vi "pump control trial.vi"(2 "Set standby speed":bool, 4 "Standby/Full speed":bool, 5 "Set standby speed":dbl=20.0 min=20.0 max=30.0 step=0.3000030517578125 format="%#.1f", 7 "VISA resource name":refnum<visa-resource-name>, 8 "Turn On/Off":bool) -> (0 "Pump controller temperature":dbl, 1 "Pump temperature":dbl, 3 "Speed":dbl, 6 "% full speed":i8)   [LabVIEW 2016]
uses:
  <vilib>/Instr/_visa.llb/VISA Configure Serial Port (Instr).vi
panel:
  out "error out 4":errorcluster
  out "error out 3":errorcluster
  out "error out":errorcluster
  out "on feedback":string
  out "off feedback":string
  out "set stb feedback":string
  out "stanby conf":string
  out "full conf":string
  out "error out 2":errorcluster
  out "Standby/Full speed 2":bool
  out "temperature feedback":string
  out "Running speed":string
  in  "baud rate (9600)":u32=9600
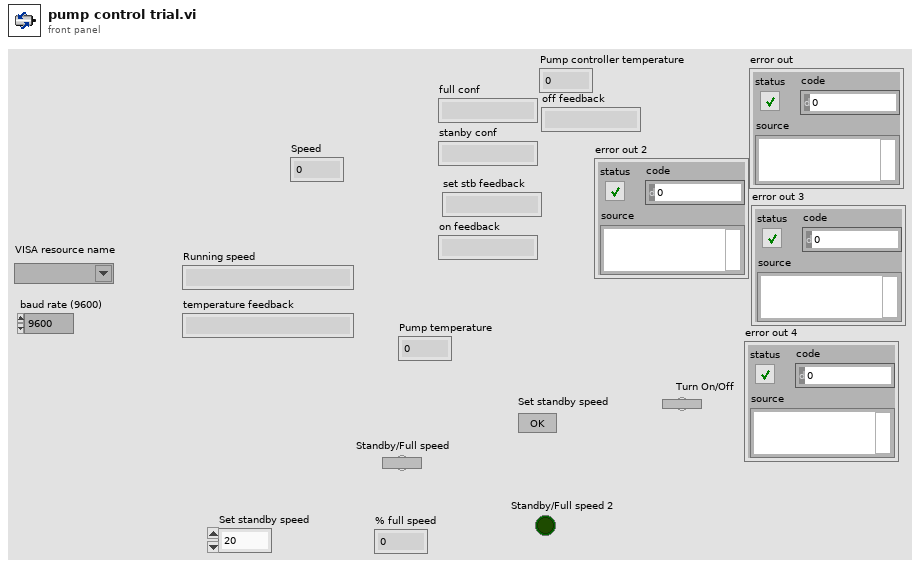
[diagram p1: front panel]
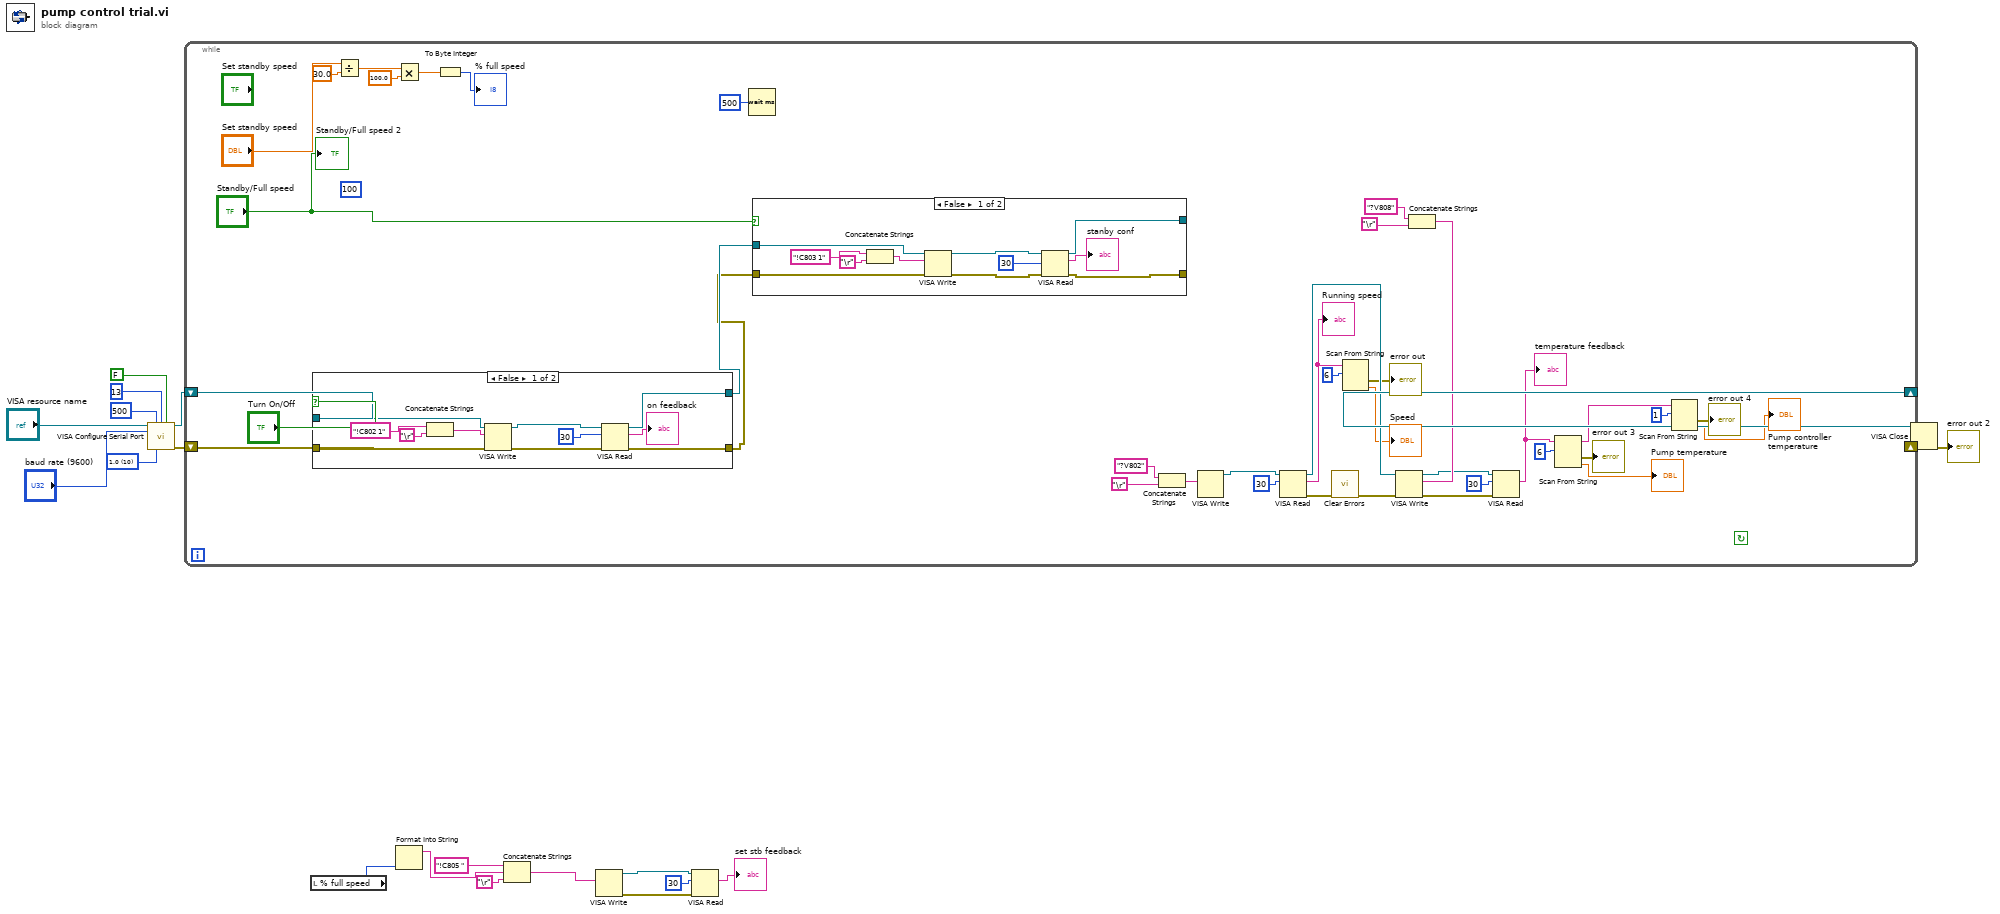
[diagram p0: block diagram]
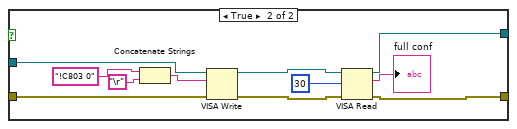
[diagram p2: hidden frame]
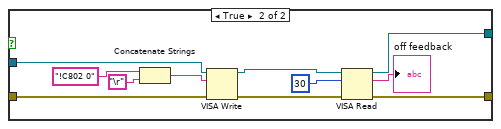
[diagram p3: hidden frame]
diagram:
  w18 = u16 10 items=["1.0"=10, "1.5"=15, "2.0"=20] ("stop bits (10: 1 bit)")
  n1 = call-poly "VISA Configure Serial Port"("VISA resource name"="VISA resource name", "timeout (10sec)"=u32 500, "termination char\n(0xA = '\\n' = LF)"=u8 13 ("termination char\n(0xA = '\\n' = LF)"), "Enable Termination\nChar (T)"=FALSE ("Enable Termination\nChar (T)"), "baud rate (9600)"="baud rate (9600)", "stop bits (10: 1 bit)"=w18) -> ("VISA resource name out"=w17:refnum<visa-resource-name>, "error out"=w16:errorcluster)  [unwired: 8 in]
  n2 = while {
    shift-right: [w61] -> w14
    shift-left: w17 -> [w28]
    shift-right: [w62] -> w13
    shift-left: w16 -> [w27]
    stop <- _ continue-if-true
    (unwired) 100
    n3 = case shown="False" "Turn On/Off" {
      tunnel: w28 -> [w99 w112]
      tunnel: w27 -> [w98 w110]
      tunnel: [w92 w108] -> w24
      tunnel: [w97 w107] -> w25
      frame False {
        n4 = Concatenate Strings("!C802 1" ("string"), "\r" ("string")) -> (w94:string)
        n5 = VISA Write(VISA resource name=w99, write buffer=w94, error in (no error)=w98) -> (VISA resource name out=w101:refnum<visa-resource-name>, error out=w100:errorcluster)  [unwired: 1 out]
        n6 = VISA Read(VISA resource name=w101, byte count=u32 30, error in (no error)=w100) -> (VISA resource name out=w97:refnum<visa-resource-name>, read buffer=→"on feedback":string, error out=w92:errorcluster)  [unwired: 1 out]
      }
      frame True {
        n7 = Concatenate Strings("!C802 0" ("string"), "\r" ("string")) -> (w104:string)
        n8 = VISA Write(VISA resource name=w112, write buffer=w104, error in (no error)=w110) -> (VISA resource name out=w111:refnum<visa-resource-name>, error out=w109:errorcluster)  [unwired: 1 out]
        n9 = VISA Read(VISA resource name=w111, byte count=u32 30, error in (no error)=w109) -> (VISA resource name out=w107:refnum<visa-resource-name>, read buffer=→"off feedback":string, error out=w108:errorcluster)  [unwired: 1 out]
      }
    }
    n10 = Divide(x="Set standby speed", y=30.0) -> (x/y=w64:dbl)
    n11 = Multiply(x=w64, y=sgl 100.0) -> (x*y=w67:dbl)
    n12 = To Byte Integer(number=w67) -> (8bit integer=→"% full speed":i8)
    n13 = Wait (ms)(milliseconds to wait=u32 500) -> ()  [unwired: 1 out]
    n14 = case shown="False" "Standby/Full speed" {
      tunnel: w25 -> [w76 w86]
      tunnel: w24 -> [w78 w85]
      tunnel: [w77 w84] -> _
      tunnel: [w74 w83] -> _
      frame False {
        n15 = Concatenate Strings("!C803 1" ("string"), "\r") -> (w73:string)
        n16 = VISA Write(VISA resource name=w76, write buffer=w73, error in (no error)=w78) -> (VISA resource name out=w75:refnum<visa-resource-name>, error out=w79:errorcluster)  [unwired: 1 out]
        n17 = VISA Read(VISA resource name=w75, byte count=u32 30, error in (no error)=w79) -> (VISA resource name out=w74:refnum<visa-resource-name>, read buffer=→"stanby conf":string, error out=w77:errorcluster)  [unwired: 1 out]
      }
      frame True {
        n18 = Concatenate Strings("!C803 0" ("string"), "\r") -> (w88:string)
        n19 = VISA Write(VISA resource name=w86, write buffer=w88, error in (no error)=w85) -> (VISA resource name out=w89:refnum<visa-resource-name>, error out=w90:errorcluster)  [unwired: 1 out]
        n20 = VISA Read(VISA resource name=w89, byte count=u32 30, error in (no error)=w90) -> (VISA resource name out=w83:refnum<visa-resource-name>, read buffer=→"full conf":string, error out=w84:errorcluster)  [unwired: 1 out]
      }
    }
    n21 = Concatenate Strings("?V802" ("write buffer"), "\r") -> (w52:string)
    n22 = VISA Write(write buffer=w52) -> (VISA resource name=w58:refnum<visa-resource-name>, error in (no error)=w59:errorcluster, VISA resource name out=w53:refnum<visa-resource-name>)  [unwired: 2 out]
    n23 = VISA Read(VISA resource name=w53, byte count=u32 30) -> (VISA resource name out=w55:refnum<visa-resource-name>, read buffer=w36:string, error out=w44:errorcluster)  [unwired: 1 in, 1 out]
    "Running speed" <- w36
    n24 = call <vilib>:"Clear Errors.vi"("error in (no error)"=w44) -> ("error out"=w33:errorcluster)  [unwired: 5 in, 1 out]
    n25 = Scan From String(input string=w36, initial scan location=u32 6) -> (error out=→"error out":errorcluster, output 1=→"Speed":dbl)  [unwired: 3 in, 2 out]
    n26 = Concatenate Strings("?V808" ("write buffer"), "\r") -> (w47:string)
    n27 = VISA Write(VISA resource name=w55, write buffer=w47, error in (no error)=w33) -> (VISA resource name out=w46:refnum<visa-resource-name>, error out=w43:errorcluster)  [unwired: 1 out]
    n28 = VISA Read(VISA resource name=w46, byte count=u32 30, error in (no error)=w43) -> (VISA resource name out=w56:refnum<visa-resource-name>, read buffer=w42:string, error out=w57:errorcluster)  [unwired: 1 out]
    "temperature feedback" <- w42
    n29 = Scan From String(input string=w42, initial scan location=u32 6) -> (remaining string=w39:string, error out=→"error out 3":errorcluster, output 1=→"Pump temperature":dbl)  [unwired: 3 in, 1 out]
    n30 = Scan From String(input string=w39, initial scan location=u32 1) -> (error out=→"error out 4":errorcluster, output 1=→"Pump controller temperature":dbl)  [unwired: 3 in, 2 out]
    "Standby/Full speed 2" <- "Standby/Full speed"
  }
  n31 = local read "% full speed"() -> (w1:i8)
  n32 = Format Into String(w1) -> (resulting string=w4:string)  [unwired: 3 in, 1 out]
  n33 = Concatenate Strings("!C805 " ("string"), w4, "\r" ("string")) -> (w6:string)
  n34 = VISA Write(write buffer=w6) -> (VISA resource name=w7:refnum<visa-resource-name>, VISA resource name out=w11:refnum<visa-resource-name>, error out=w2:errorcluster)  [unwired: 1 in, 1 out]
  n35 = VISA Read(VISA resource name=w11, byte count=u32 30, error in (no error)=w2) -> (VISA resource name out=w12:refnum<visa-resource-name>, read buffer=→"set stb feedback":string, error out=w8:errorcluster)  [unwired: 1 out]
  n36 = VISA Close(VISA resource name=w14, error in (no error)=w13) -> (error out=→"error out 2":errorcluster)
